vi "Get Main.Limitation.vi"(0 "Main":string="0", 1 "VI Ref":refnum<vi>, 2 "CMD":T2(ring)=enum."Read", 5 "Order By":T1, 9 "VariableName":string, 11 "error in (no error)":errorcluster, 12 "Alarm?":bool=TRUE) -> (3 "Unit":string, 4 "Data-DBL":cluster{"Max":dbl, "Min":dbl}, 6 "Data-String":cluster{"Max":string, "Min":string}, 10 "Limitation Table":string[](array[string]), 14 "Result Set":string[][](array[string]), 15 "error out":errorcluster)   [LabVIEW 2017, in "SQLite.lvclass"]
doc: "get Limitation Data.\n2015-11-03 10:56:51\n蒋松\njiangsong@outlook.com"
uses:
  SQLite.lvclass
  Order By.ctl
  SQLiteFileName.ctl
  TabelFullName.ctl
  <vilib>/Utility/error.llb/Trim Whitespace.vi
  <userlib>/LabSQL/LabSQL.lvlib
  <userlib>/sushu/sushu.lvlib
panel:
  out "Select SQL CMD":string
  # "Initialize\nRead\nWrite\nUnInitialize"
  # "TorqueAnglePrecision"
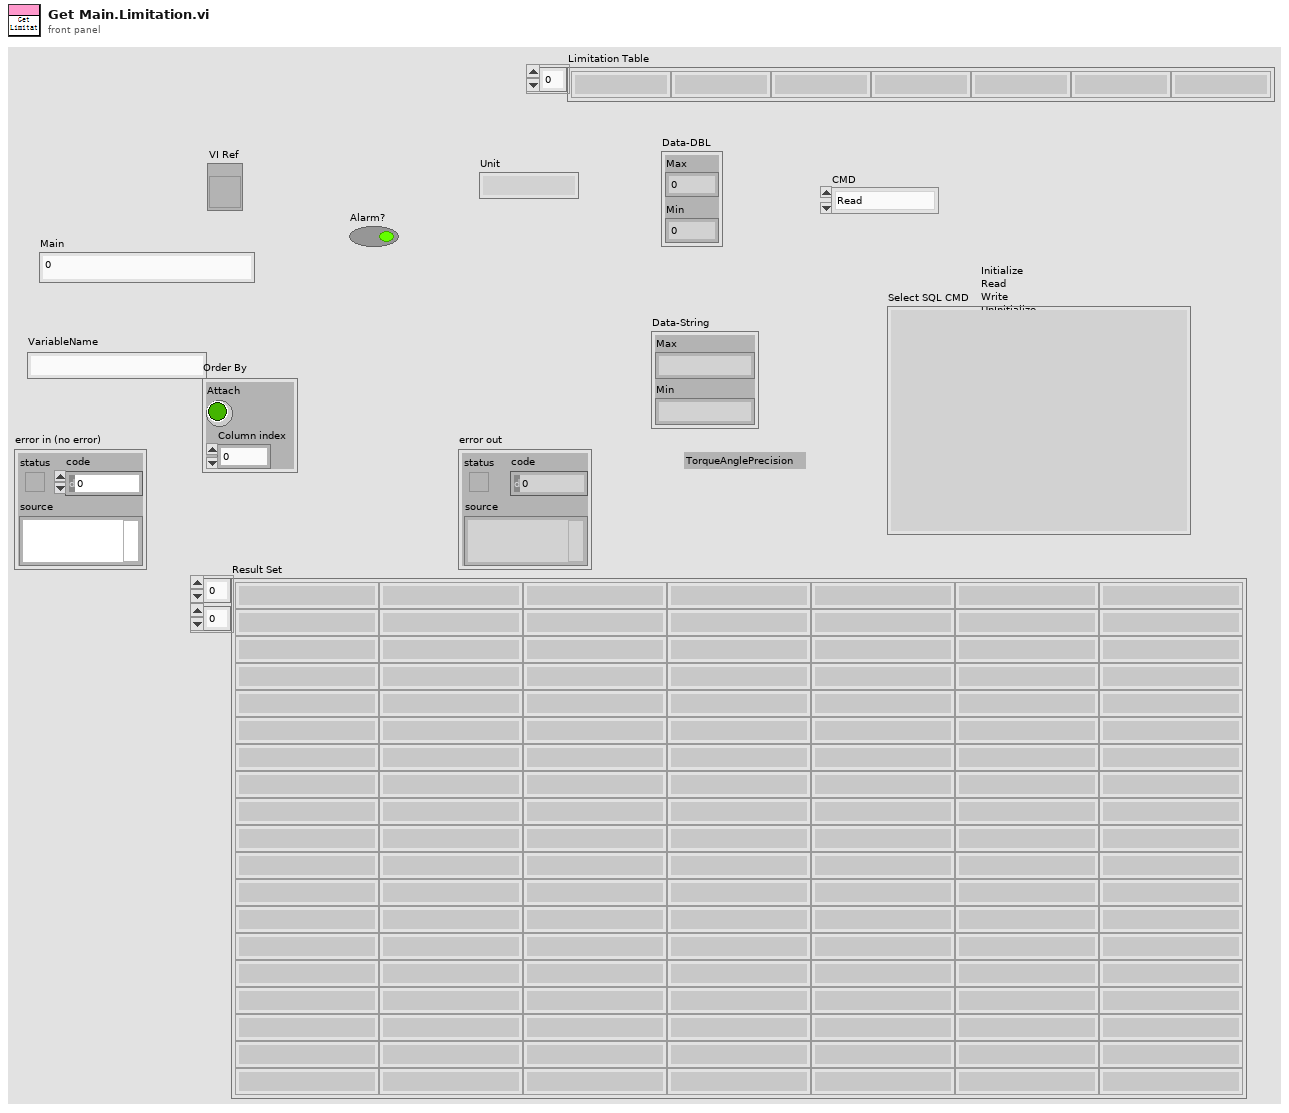
[diagram p1: front panel]
types:
  T1 = typedef "SQLite.lvclass/Order By.ctl" = cluster{"Attach":bool, "Column index":i32}
  T2 = enum16{"Initialize", "Read", "Write", "UnInitialize"}
  T3 = typedef "SQLite.lvclass/TabelFullName.ctl" = string
  T4 = typedef "SQLite.lvclass/SQLiteFileName.ctl" = string
  T5 = cluster{"Current VI Reference":refnum<vi>, "Close Panel on Exit?":bool}
  T6 = cluster{"Core":cluster{"Current VI Reference":refnum<vi>, "Close Panel on Exit?":bool}, "VI Name":string}
  T7 = enum32{"invalid app kind", "Development System", "Run Time System", "Student Edition", "Embedded LabVIEW", "Evaluation", "Custom"}
  T8 = enum32{"Invalid", "Standard", "Closed", "Hidden", "Minimized", "Maximized"}
  T9 = enum16{"Other", "SQL2008", "SQLite", "Access", "MySQL"}
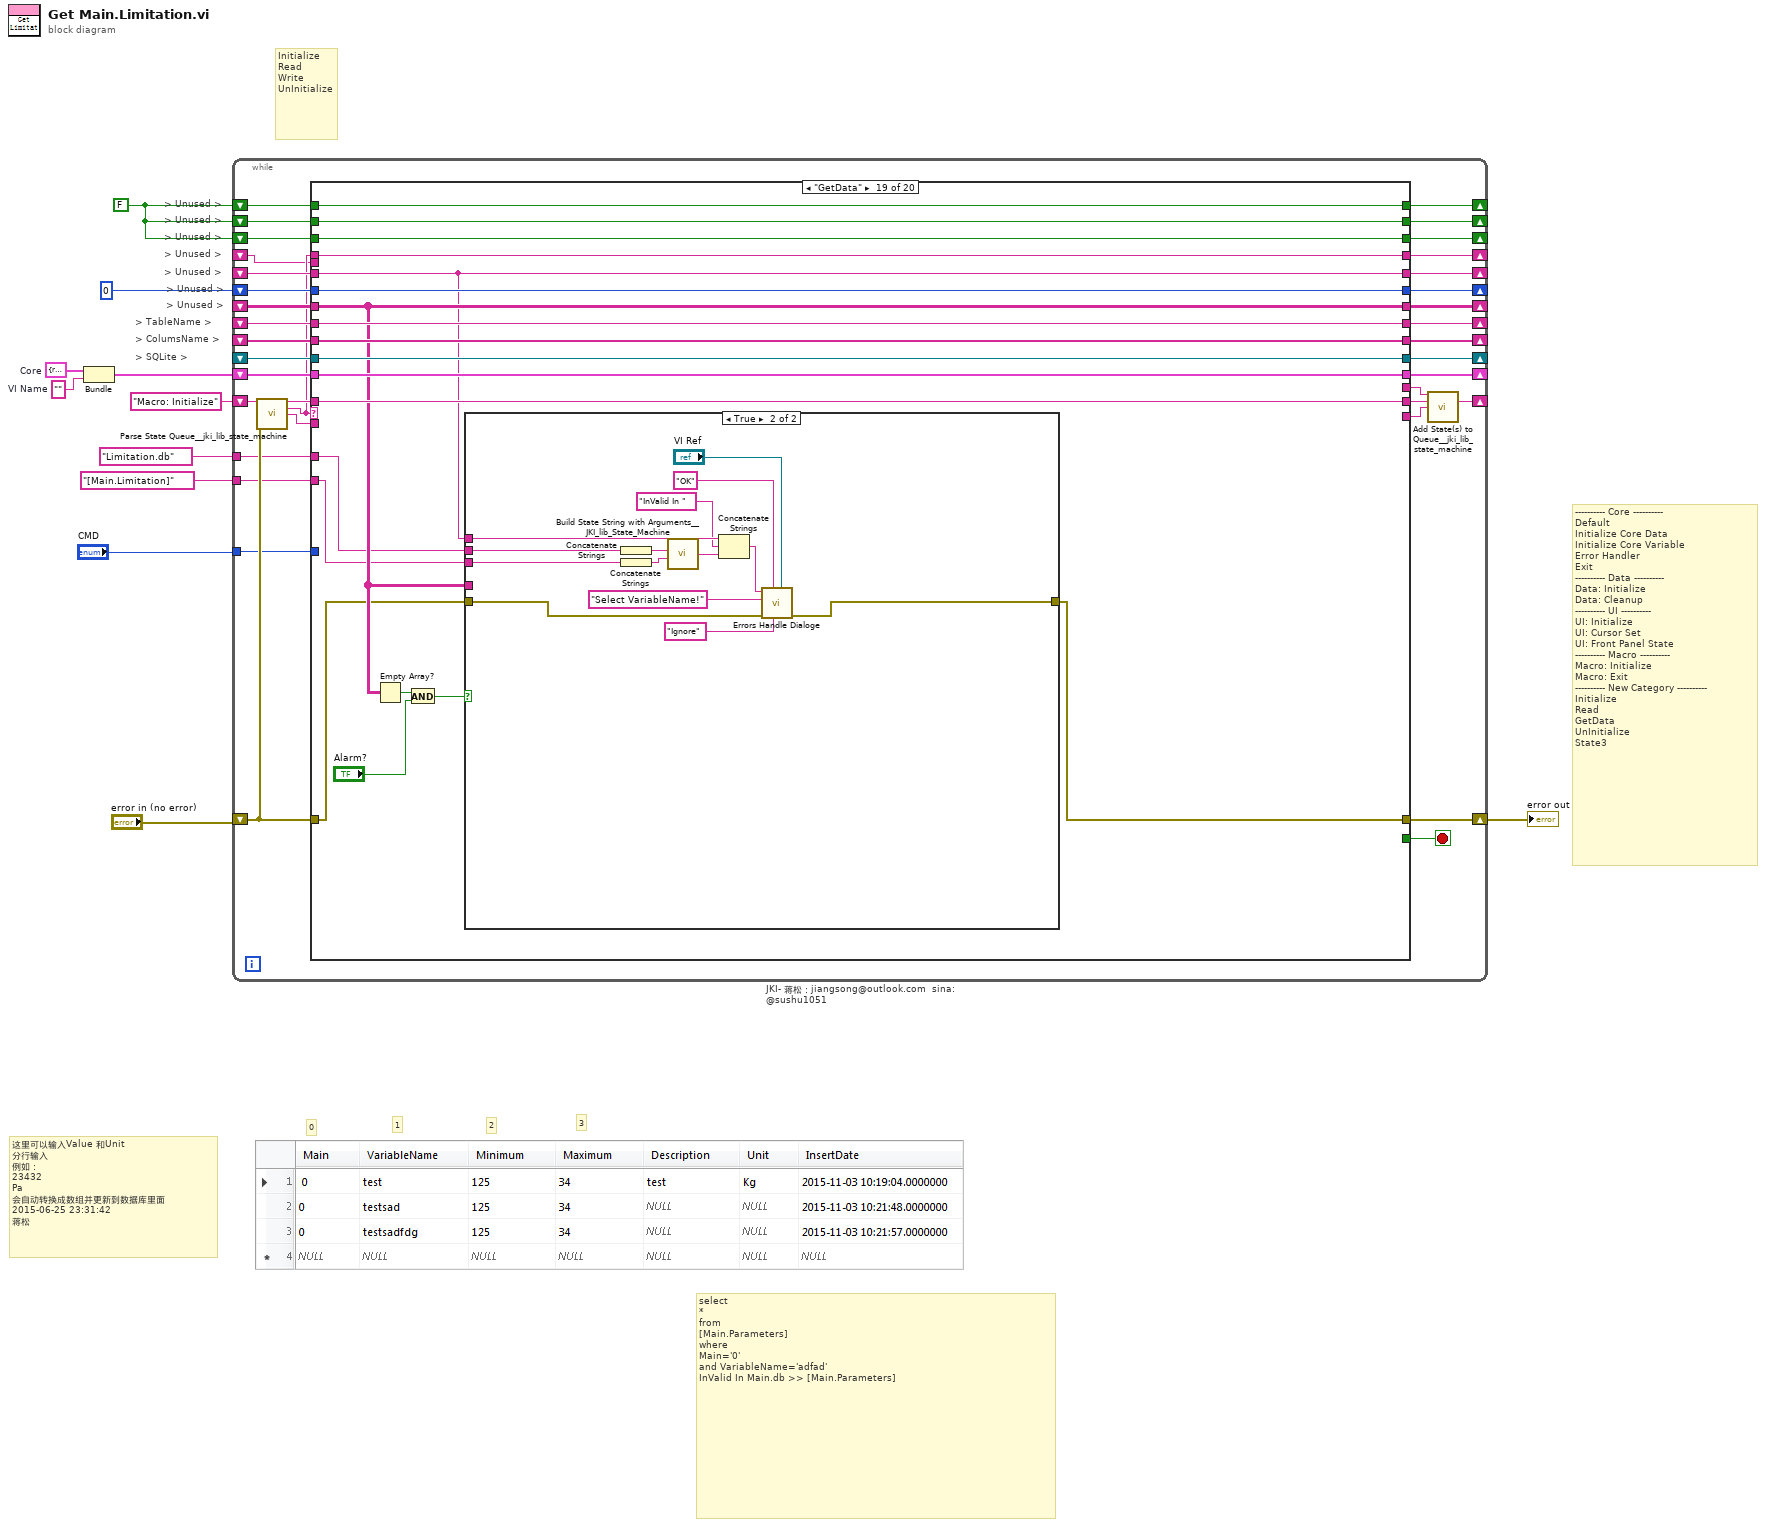
[diagram p0: block diagram]
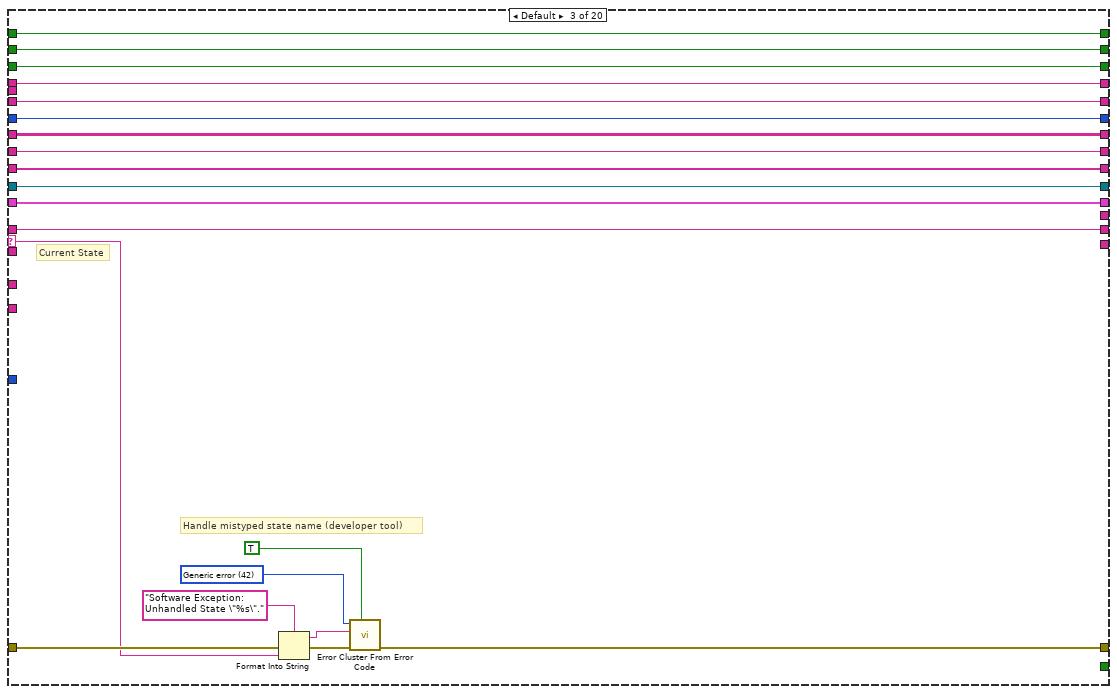
[diagram p4: hidden frame]
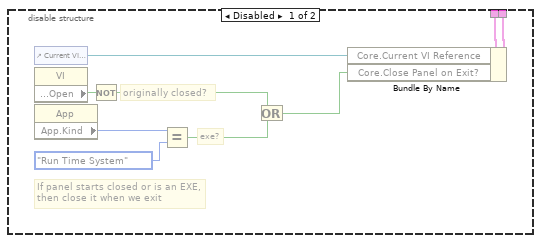
[diagram p6: hidden frame]
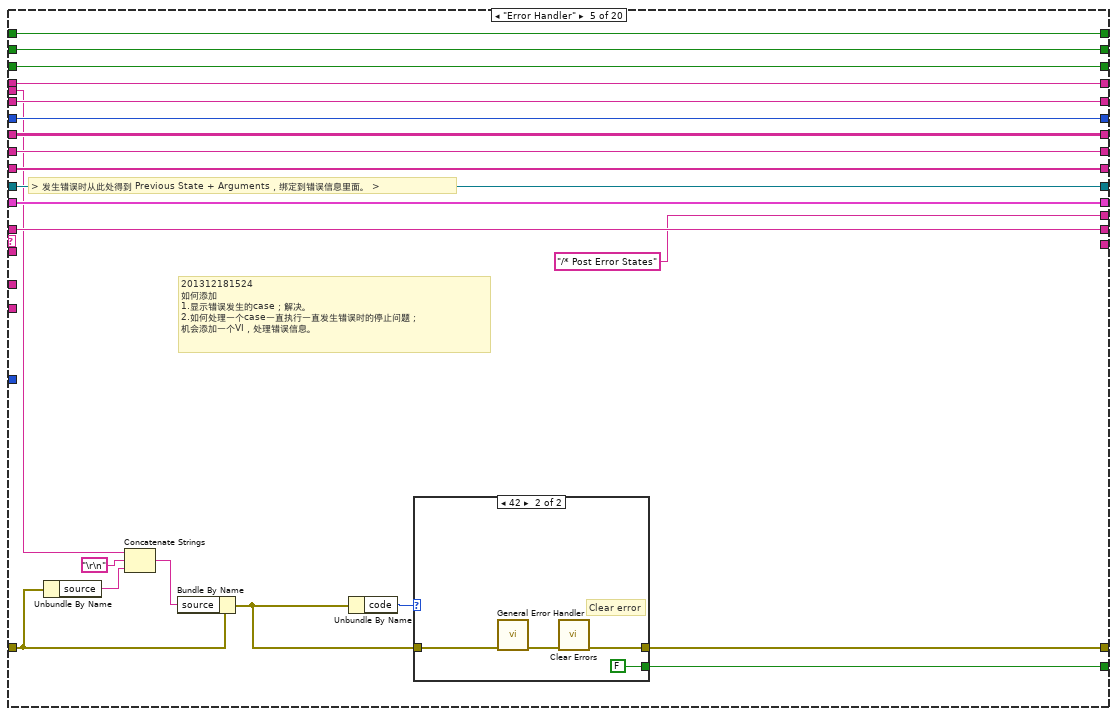
[diagram p7: hidden frame]
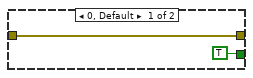
[diagram p8: hidden frame]
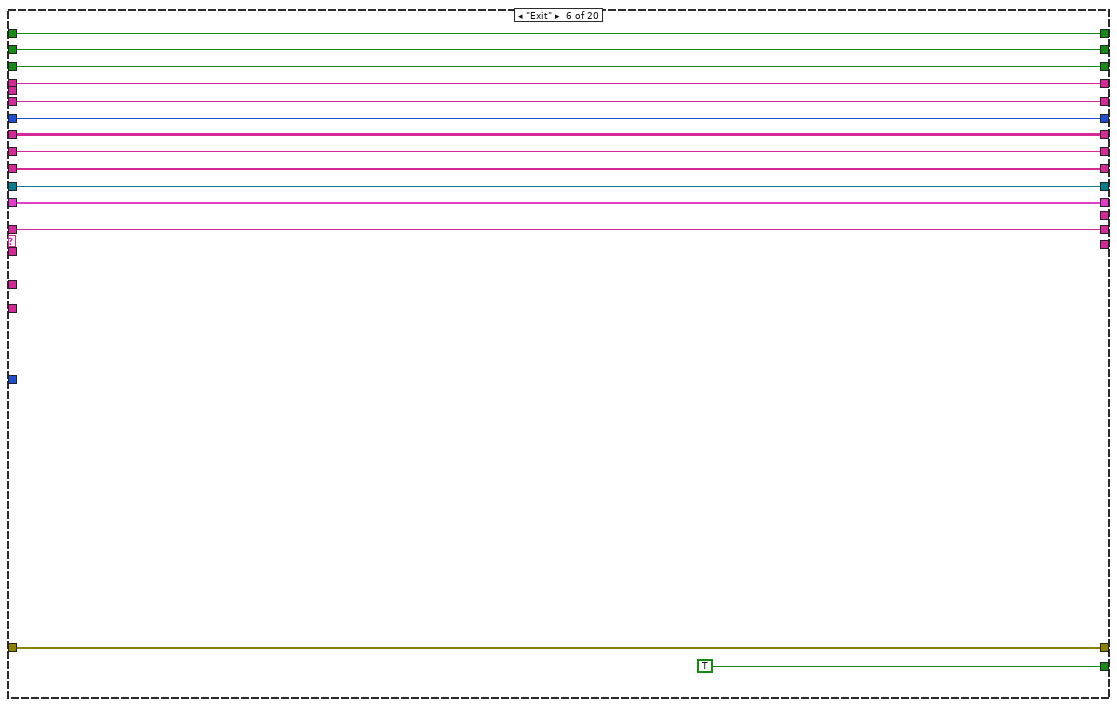
[diagram p9: hidden frame]
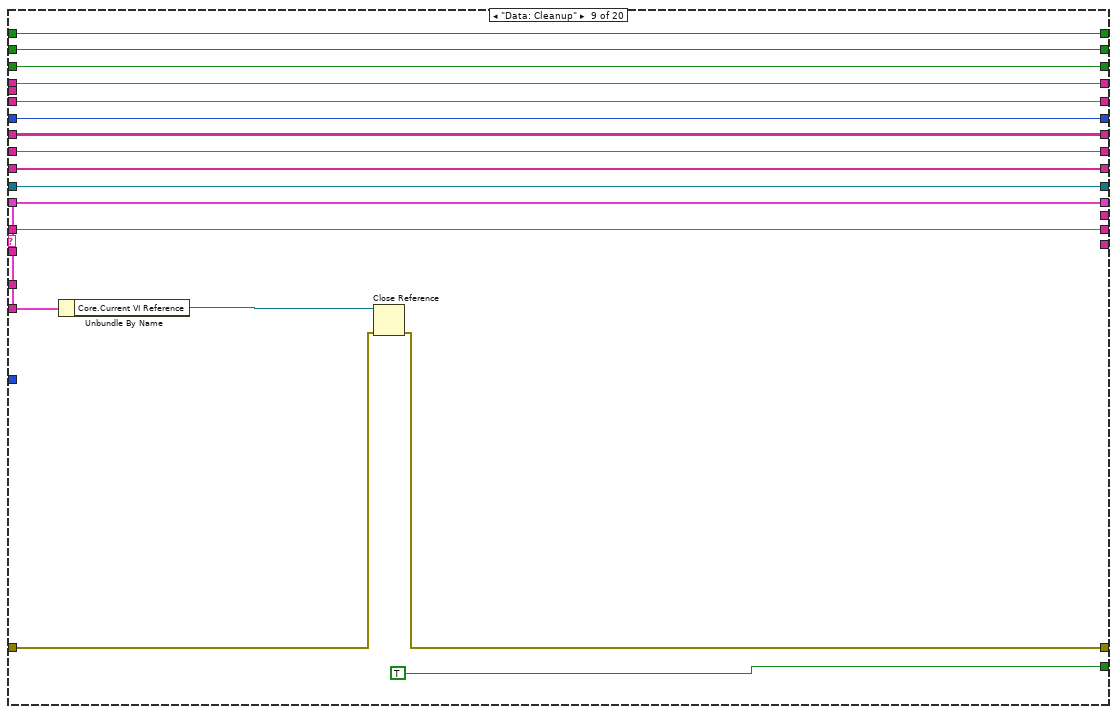
[diagram p12: hidden frame]
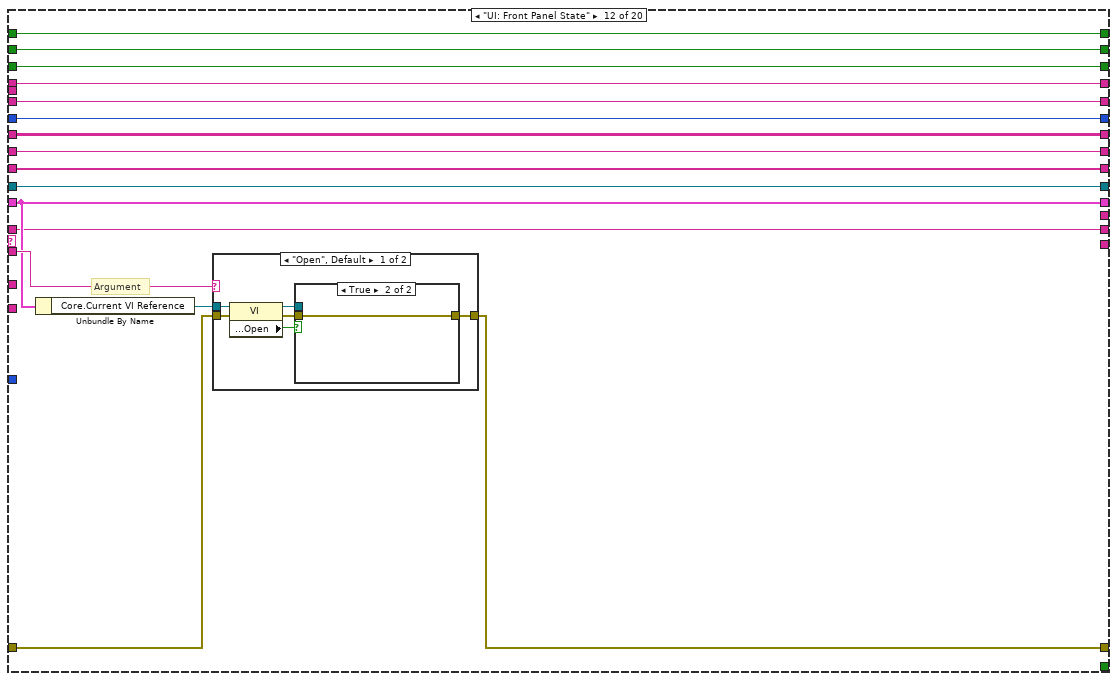
[diagram p15: hidden frame]
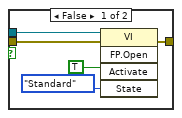
[diagram p16: hidden frame]
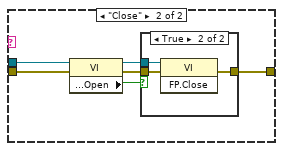
[diagram p17: hidden frame]
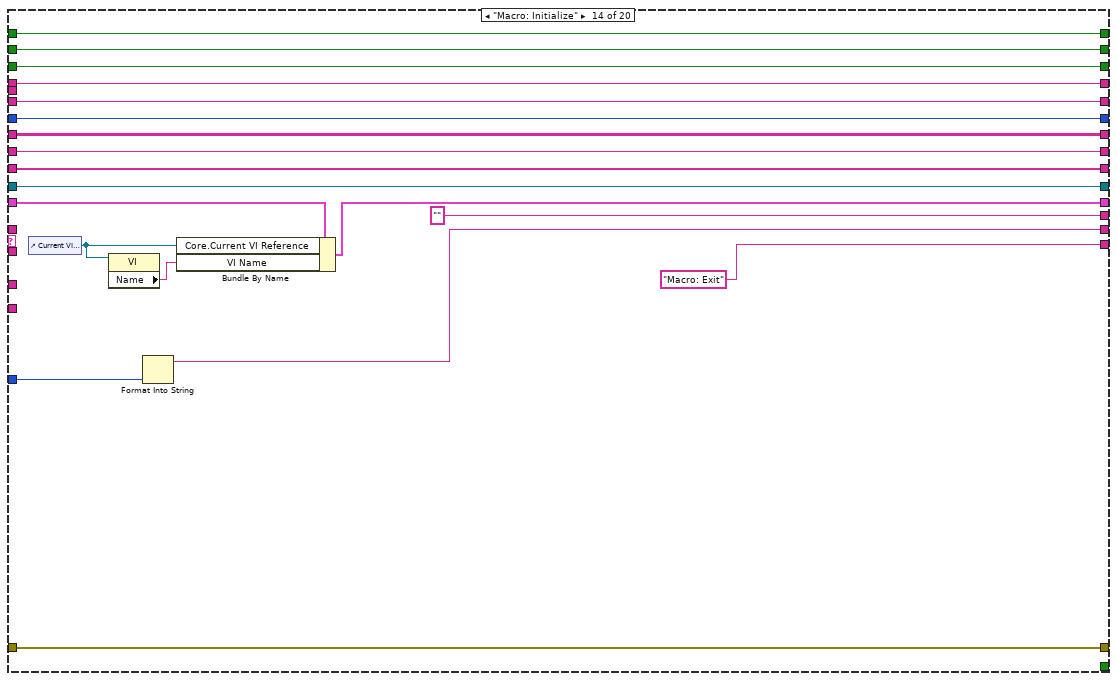
[diagram p20: hidden frame]
diagram:
  w11 = ""  # VI Name
  w10 = T5 {"Current VI Reference"=refnum, "Close Panel on Exit?"=FALSE}  # Core
  w3 = FALSE
  # "Initialize\nRead\nWrite\nUnInitialize"
  # "> Unused >"
  # "> Unused >"
  # "> Unused >"
  # "> Unused >"
  # "> Unused >"
  # "> Unused >"
  # "> SQLite >"
  # "> ColumsName >"
  # "> TableName >"
  # "> Unused >"
  # "---------- Core ----------\nDefault\nInitialize Core Data\nInitialize Core Variable\nError Handler\nExit\n---------- Data ----------\nData: Initialize\nData: Cleanup\n---------- UI ----------\nUI: Initialize\nUI: Cursor Set\nUI: Front Panel State\n---------- Macro ----------\nMacro: Initialize\nMacro: Exit\n---------- New Category ----------\nInitialize\nRead\nGetData\nUnInitialize\nState3"
  # "3"
  # "2"
  # "1"
  # "0"
  # "select\n*\nfrom\n[Main.Parameters]\nwhere\nMain='0'\nand VariableName='adfad'\nInValid In Main.db >> [Main.Parameters]"
  # "这里可以输入Value 和Unit\n分行输入\n例如：\n23432\nPa\n会自动转换成数组并更新到数据库里面\n2015-06-25 23:31:42\n蒋松"
  n1 = Bundle("Core"=w10, "VI Name"=w11) -> (w9:T6)  [unwired: 1 in]
  n2 = while "JKI- 蒋松：jiangsong@outlook.com  sina: @sushu1051" {
    shift-right: [w45] -> w5
    shift-left: "error in (no error)" -> [w43]
    shift-right: [w32] -> _
    shift-left: "Macro: Initialize" -> [w33]
    shift-right: [w39] -> _
    shift-left: _ -> [w41]
    shift-right: [w40] -> _
    shift-left: _ -> [w42]
    shift-right: [w34] -> _
    shift-left: w9 -> [w37]
    shift-right: [w35] -> _
    shift-left: _ -> [w28]
    shift-right: [w36] -> _
    shift-left: _ -> [w38]
    shift-right: [w27] -> _
    shift-left: 0 -> [w26]
    shift-right: [w20] -> _
    shift-left: w3 -> [w18]
    shift-right: [w19] -> _
    shift-left: w3 -> [w17]
    shift-right: [w22] -> _
    shift-left: _ -> [w23]
    shift-right: [w21] -> _
    shift-left: _ -> [w12]
    shift-right: [w24] -> _
    shift-left: w3 -> [w25]
    tunnel: "CMD" -> [w16]
    tunnel: T4 "Limitation.db" ("SQLiteFileName") -> [w15]
    tunnel: T3 "[Main.Limitation]" ("TabelFullName") -> [w14]
    stop <- w44 stop-if-true
    n3 = call <vilib>:"Parse State Queue__jki_lib_state_machine.vi"("State Queue"=w33, "Error In (no error)"=w43) -> ("Remaining States"=w47:string, "Current State"=w13:string, "Arguments"=w46:string)  [unwired: 10 in, 1 out]
    n4 = case shown="\"GetData\"" w13 {
      selector: w13 -> [_ _ w81 _ _ _ _ _ _ _ _ _ _ _ _ _ _ w358 _ _]
      tunnel: w47 -> [w60 w67 w80 w100 w131 w152 w166 w180 w193 w208 w221 w234 w272 _ w305 w322 w348 w383 w420 w469]
      tunnel: w46 -> [_ _ _ _ _ _ _ _ _ _ _ w237 _ _ _ _ _ _ _ _]
      tunnel: [w59 w73 w82 w104 w125 w154 w168 w182 w195 w210 w223 w238 w274 w294 w312 w325 w329 w353 w405 w455] -> w45
      tunnel: w43 -> [w59 w73 w83 w104 w135 w154 w168 w182 w196 w210 w223 w239 w274 w294 w312 w325 w329 w353 w406 w456]
      tunnel: [w60 w67 w80 w100 w131 w152 w166 w180 w193 w208 w221 w234 w272 w280 w305 w322 w348 w383 w420 w469] -> w31
      tunnel: [_ _ _ _ w124 TRUE _ _ TRUE _ _ _ _ _ _ _ _ _ _ _] -> w44
      tunnel: w42 -> [w58 w72 w93 w107 w139 w159 w172 w185 w201 w214 w227 w243 w278 w297 w315 w328 w347 _ w407 w468]
      tunnel: w41 -> [w57 w71 w92 w106 w138 w158 w171 w184 w200 w213 w226 w242 w277 w296 w314 w327 _ w363 w419 w467]
      tunnel: [w58 w72 w93 w107 w139 w159 w172 w185 w201 w214 w227 w243 w278 w297 w315 w328 w347 w354 w407 w468] -> w40
      tunnel: [w57 w71 w92 w106 w138 w158 w171 w184 w200 w213 w226 w242 w277 w296 w314 w327 w330 w363 w419 w467] -> w39
      tunnel: w38 -> [w56 w70 w91 w105 w137 w157 w170 w183 w199 w212 w225 w241 w276 w295 w313 w326 _ w364 w418 w466]
      tunnel: w28 -> [w54 w68 w90 w101 w129 w153 w167 w181 w194 w209 w222 w235 w273 w293 w306 w323 _ w357 w417 w458]
      tunnel: w37 -> [w55 w69 w89 w103 w136 w156 w169 w173 w197 w211 w224 w236 w275 w282 w307 w324 w346 w382 w416 w465]
      tunnel: [w56 w70 w91 w105 w137 w157 w170 w183 w199 w212 w225 w241 w276 w295 w313 w326 w332 w364 w418 w466] -> w36
      tunnel: [w54 w68 w90 w101 w129 w153 w167 w181 w194 w209 w222 w235 w273 w293 w306 w323 w334 w356 w417 w457] -> w35
      tunnel: [w55 w69 w89 w102 w136 w156 w169 w173 w197 w211 w224 w236 w275 w281 w307 w324 w346 w382 w416 w465] -> w34
      tunnel: [_ _ _ _ "/* Post Error States" _ _ _ _ _ _ _ _ "" w304 _ _ w360 _ _] -> w30
      tunnel: [_ _ _ _ _ _ _ _ _ _ _ _ _ "Macro: Exit" _ _ _ _ _ _] -> w29
      tunnel: w26 -> [w53 w66 w79 w99 w128 w151 w165 w179 w192 w207 w220 w233 w271 w292 w303 w321 w345 w361 w415 w464]
      tunnel: [w53 w66 w79 w99 w128 w151 w165 w179 w192 w207 w220 w233 w271 w292 w303 w321 w345 w362 w415 w464] -> w27
      tunnel: w17 -> [w51 w64 w77 w97 w122 w149 w163 w177 w190 w205 w218 w231 w269 w288 w301 w319 w340 w380 w414 w463]
      tunnel: w18 -> [w50 w63 w76 w96 w121 w148 w162 w176 w189 w204 w217 w230 w268 w287 w300 w318 w341 w379 w413 w462]
      tunnel: [w51 w64 w77 w97 w122 w149 w163 w177 w190 w205 w218 w231 w269 w288 w301 w319 w340 w380 w414 w463] -> w19
      tunnel: [w50 w63 w76 w96 w121 w148 w162 w176 w189 w204 w217 w230 w268 w287 w300 w318 w341 w379 w413 w462] -> w20
      tunnel: w13 -> [w49 w62 w75 w95 w120 w147 w161 w175 w188 w203 w216 w229 w267 w286 w299 w317 w342 w378 w412 w461]
      tunnel: w23 -> [w48 w61 w74 w94 w119 w146 w160 w174 w187 w202 w215 w228 w266 w285 w298 w316 w343 _ w402 w460]
      tunnel: [w49 w62 w75 w95 w120 w147 w161 w175 w188 w203 w216 w229 w267 w286 w299 w317 w342 w378 w412 w461] -> w21
      tunnel: [w48 w61 w74 w94 w119 w146 w160 w174 w187 w202 w215 w228 w266 w285 w298 w316 w343 w355 w402 w460] -> w22
      tunnel: w25 -> [w52 w65 w78 w98 w123 w150 w164 w178 w191 w206 w219 w232 w270 w289 w302 w320 w344 w381 w411 w459]
      tunnel: [w52 w65 w78 w98 w123 w150 w164 w178 w191 w206 w219 w232 w270 w289 w302 w320 w344 w381 w411 w459] -> w24
      tunnel: w16 -> [_ _ _ _ _ _ _ _ _ _ _ _ _ w279 _ _ _ _ _ _]
      tunnel: w15 -> [_ _ _ _ _ _ _ _ _ _ _ _ _ _ _ _ w333 _ w404 _]
      tunnel: w14 -> [_ _ _ _ _ _ _ _ _ _ _ _ _ _ _ _ w331 _ w403 _]
      tunnel: w12 -> [_ _ _ _ w118 _ _ _ _ _ _ _ _ _ _ _ _ _ _ _]
      frame "Idle" {
      }
      frame "---------- Core ----------" {
      }
      frame Default {
        w85 = 42 items=["No error", "Argument error", "Memory is full", "Out of zone", "End of file", "File already open", "Generic file I/O error", "File not found", "File permission error", "Disk is full", "Duplicate path", "Too many files open", "System feature not enabled", "Resource file not found", "Cannot add resource", "Resource not found", "Image not found", "Image memory error", "Pen does not exist", "Config type invalid", "Config token not found", "Config parse error", "Config memory error", "Bad external code format", "Bad external code offset", "External code not present", "Null window", "Destroy window error", "Null menu", "Print aborted", "Bad print record", "Print driver error", "Windows error during printing", "Memory error during printing", "Print dialog error", "Generic print error", "Invalid device refnum", "Device not found", "Device parameter error", "Device unit error", "Cannot open device", "Device call aborted", "Generic error", "Cancelled by user", "Object ID too low", "Object ID too high", "Object not in heap", "Unknown heap", "Unknown object (invalid DefProc)", "Unknown object (DefProc not in table)", "Message out of range", "Invalid (null) method", "Unknown message", "Manager call not supported", "Bad address", "Network operation in progress", "Network operation timed out", "Connection is busy", "Network attribute not supported", "Network error", "Address in use", "System out of memory", "Connection aborted", "Connection refused", "Not connected", "Already connected", "Connection closed", "Initialization error (interapplication manager)", "Bad occurrence", "Wait on unbound occurrence handler", "Occurrence queue overflow", "Datalog type conflict", "Unused", "Unrecognized type (interapplication manager)", "Memory corrupt", "Failed to make temporary DLL", "Old CIN version", "Drag socket not found", "Failed to load drop-object", "Failed to register OLE object", "Failed to release OLE object", "Format specifier type mismatch", "Unknown format specifier", "Too few format specifiers", "Too many format specifiers", "Scan failed", "Newer CIN version", "Error converting to variant", "Runtime menu error", "Password tampered", "Variant attribute not found", "Incompatible variant data type", "Event data is not available", "Event Store is not present", "Occurrence is not found", "Event Queue is not created", "Event info is not available", "Refnum passed is NULL", "Error retrieving Class GUID", "Error retrieving CoClass GUID", "Error retrieving TypeLib GUID.", "Bad built application magic bytes.", "Specific driver is different from the specific driver associated with the Logical Name.", "There is no session opened to the class driver.", "Max Error", "MAX - Error with config objects", "MAX - Error loading configuration", "MAX - Group not supported"]
        # "Current State"
        # "Handle mistyped state name (developer tool)"
        n5 = Format Into String(format string="Software Exception: Unhandled State \"%s\"." ("message"), error in=w83, w81) -> (resulting string=w86:string, error out=w87:errorcluster)  [unwired: 1 in]
        n6 = call <vilib>:"Error Cluster From Error Code.vi"("show call chain? (False)"=TRUE, "error in (no error)"=w87, "error message (\"\")"=w86, "error code (0)"=w85) -> ("error out"=w82:errorcluster)  [unwired: 5 in]
      }
      frame "Initialize Core Data" {
        n7 = disable-structure shown="Enabled" {
          disable-tunnel: w103 -> [w109 w117]
          disable-tunnel: [w108 w117] -> w102
          frame Disabled {
            # "originally closed?"
            # "exe?"
            # "If panel starts closed or is an EXE, then close it when we exit"
            n8 = control-ref of="Current VI Reference"() -> (w116:refnum<vi>)
            n9 = property class="VI"() -> ("Front Panel.Open"=w110:bool)  [unwired: 2 in, 2 out]
            n10 = property class="App"() -> ("App.Kind"=w111:T7)  [unwired: 2 in, 2 out]
            n11 = Not(x=w110) -> (.not. x?=w113:bool)
            n12 = Equal?(x=w111, y=T7."Run Time System" ("Application:Kind")) -> (x = y?=w114:bool)
            n13 = Or(x=w113, y=w114) -> (x .or. y?=w115:bool)
            n14 = Bundle By Name(cluster=w109, "Core.Current VI Reference"=w116, "Core.Close Panel on Exit?"=w115) -> (w108:T6)
          }
          frame Enabled {
          }
        }
      }
      frame "Error Handler" {
        # "> 发生错误时从此处得到 Previous State + Arguments，绑定到错误信息里面。 >"
        # "201312181524\n如何添加\n1.显示错误发生的case；解决。\n2.如何处理一个case一直执行一直发生错误时的停止问题；\n机会添加一个VI，处理错误信息。"
        # "Clear error"
        n15 = Unbundle By Name(w135) -> ("source"=w133:string)
        n16 = Concatenate Strings(w118, "\r\n", w133) -> (w132:string)
        n17 = Bundle By Name(cluster=w135, "source"=w132) -> (w126:errorcluster)
        n18 = Unbundle By Name(w126) -> ("code"=w127:i32)
        n19 = case shown="42" w127 {
          tunnel: [TRUE FALSE] -> w124
          tunnel: w126 -> [w141 w144]
          tunnel: [w141 w142] -> w125
          frame 0, Default {
          }
          frame 42 {
            n20 = call <vilib>:"General Error Handler.vi"("error in (no error)"=w144) -> ("error out"=w143:errorcluster)  [unwired: 10 in, 4 out]
            n21 = call <vilib>:"Clear Errors.vi"("error in (no error)"=w143) -> ("error out"=w142:errorcluster)  [unwired: 5 in, 1 out]
          }
        }
      }
      frame "Exit" {
      }
      frame "---------- Data ----------" {
      }
      frame "Data: Initialize" {
      }
      frame "Data: Cleanup" {
        n22 = Unbundle By Name(w197) -> ("Core.Current VI Reference"=w198:refnum<vi>)
        n23 = Close Reference(reference=w198, error in (no error)=w196) -> (error out=w195:errorcluster)
      }
      frame "---------- UI ----------" {
      }
      frame "UI: Initialize" {
      }
      frame "UI: Front Panel State" {
        # "Argument"
        n24 = Unbundle By Name(w236) -> ("Core.Current VI Reference"=w240:refnum<vi>)
        n25 = case shown="\"Open\", Default" w237 {
          tunnel: w239 -> [w247 w260]
          tunnel: [w249 w261] -> w238
          tunnel: w240 -> [w248 w258]
          frame "Open", Default {
            n26 = property class="VI"(reference=w248, error in=w247) -> (reference out=w245:refnum<vi>, error out=w246:errorcluster, "Front Panel.Open"=w244:bool)
            n27 = case shown="True" w244 {
              tunnel: [w252 w255] -> w249
              tunnel: w246 -> [w251 w255]
              tunnel: w245 -> [w250 _]
              frame False {
                n28 = invoke class="VI" method="FP.Open"(reference=w250, error in=w251, "Activate"=TRUE, "State"=T8."Standard") -> (error out=w252:errorcluster)  [unwired: 1 in, 4 out]
              }
              frame True {
              }
            }
          }
          frame "Close" {
            n29 = property class="VI"(reference=w258, error in=w260) -> (reference out=w257:refnum<vi>, error out=w259:errorcluster, "Front Panel.Open"=w256:bool)
            n30 = case shown="True" w256 {
              tunnel: [w262 w265] -> w261
              tunnel: w259 -> [w262 w264]
              tunnel: w257 -> [_ w263]
              frame False {
              }
              frame True {
                n31 = invoke class="VI" method="FP.Close"(reference=w263, error in=w264) -> (error out=w265:errorcluster)  [unwired: 1 in, 2 out]
              }
            }
          }
        }
      }
      frame "---------- Macro ----------" {
      }
      frame "Macro: Initialize" {
        n32 = control-ref of="Current VI Reference"() -> (w283:refnum<vi>)
        n33 = property class="VI"(reference=w283) -> ("Name"=w284:string)  [unwired: 1 in, 2 out]
        n34 = Format Into String(w279) -> (resulting string=w280:string)  [unwired: 3 in, 1 out]
        n35 = Bundle By Name(cluster=w282, "Core.Current VI Reference"=w283, "VI Name"=w284) -> (w281:T6)
      }
      frame "Macro: Exit" {
        n36 = Unbundle By Name(w307) -> ("Core.Close Panel on Exit?"=w308:bool)
        n37 = Select(t="UI: Front Panel State >> Close", s=w308, f="") -> ()  [unwired: 1 out]
        n38 = call <vilib>:"Add State(s) to Queue__jki_lib_state_machine.vi"("State(s) at Back (\"\")"="Data: Cleanup\nExit") -> ("States Out"=w304:string)  [unwired: 14 in]
      }
      frame "---------- New Category ----------" {
      }
      frame "Initialize" {
        n39 = Concatenate Strings(w331) -> (w330:string)
        n40 = call "SQLite File Path.vi"("SQLiteFileName"=w333, "SQLite in"=refnum<class "SQLite.lvclass"> refnum ("SQLite.lvclass")) -> ("string"=w337:string, "SQLite out"=w339:refnum<class "SQLite.lvclass">)  [unwired: 7 in, 1 out]
        n41 = call-dynamic "Open Connection.vi"("ConnectionString"=w337, "HostDB in"=w339) -> ("error out"=w336:errorcluster, "HostDB out"=w335:refnum<class "SQLite.lvclass">)  [unwired: 8 in]
        n42 = call-dynamic "Get Table Columns Name.vi"("error in (no error)"=w336, "TableName"=w330, "HostDB in"=w335) -> ("ColunmsList"=w332:string[], "HostDB out"=w334:refnum<class "SQLite.lvclass">)  [unwired: 4 in, 3 out]
      }
      frame "Read" {
        n43 = Empty String/Path?(string/path="VariableName") -> (empty?=w375:bool)
        n44 = Unbundle By Name("Order By") -> ("Attach"=w368:bool, "Column index"=w367:i32)
        n45 = Build Array("Main") -> (w371:string[])
        n46 = Build Array("Main", "VariableName") -> (w373:string[])
        n47 = Select(t=w371, s=w375, f=w373) -> (s? t:f=w370:string[])
        n48 = Array Size(array=w370) -> (size(s)=w369:i32)
        n49 = Array Subset(array=w364, index=0, length=w369) -> (w377:string[])
        n50 = Index Array(array=w364, index=w367) -> (element=w366:string)
        n51 = call <userlib>:"SQL_Select From DB Table.vi"("DB Type"=T9."SQLite", "ColumnsValue"=w370, "ColumnsNameList"=w377, "TableName"=w363) -> ("Select SQL CMD"=w365:string)  [unwired: 7 in]
        "Select SQL CMD" <- w365
        n52 = case shown="True" w368 {
          tunnel: w365 -> [w395 w400]
          tunnel: w366 -> [_ w398]
          tunnel: [w395 w396] -> w355
          frame False {
          }
          frame True {
            n53 = Concatenate Strings(w400, "\r", "order by cast (" ("string"), w398, " as unsigned)" ("string")) -> (w396:string)
          }
        }
        n54 = call-dynamic "SQL Execute.vi"("error in (no error)"=w353, "Return Data (T)"=TRUE, "Command Text"=w355, "HostDB in"=w357) -> ("error out"=w352:errorcluster, "Table Control"=w354:string[][], "HostDB out"=w356:refnum<class "SQLite.lvclass">)  [unwired: 3 in, 2 out]
        n55 = case shown="Error" w352 {
          tunnel: w352 -> [_ w394]
          tunnel: w361 -> [_ w393]
          tunnel: [w384 w390] -> w360
          tunnel: "GetData" ("f") -> [w384 w389]
          tunnel: w358 -> [_ w386]
          frame No Error {
          }
          frame Error {
            (unwired) 7 ("y")
            n56 = Unbundle By Name(w394) -> ("status"=w385:bool)
            n57 = Equal To 0?(x=w393) -> (x = 0?=w392:bool)
            n58 = And(x=w385, y=w392) -> (x .and. y?=w391:bool)
            n59 = call <vilib>:"Add State(s) to Queue__jki_lib_state_machine.vi"("State(s) in Front (\"\")"="Initialize" ("Remaining States"), "State(s) in (\"\")"=w386) -> ("States Out"=w387:string)  [unwired: 13 in]
            n60 = Select(t=w387, s=w391, f=w389) -> (s? t:f=w390:string)
          }
        }
        n61 = Increment(x=w361) -> (x+1=w362:i32)
      }
      frame "GetData" {
        n62 = Empty Array?(array=w407) -> (empty?=w409:bool)
        n63 = And(x=w409, y="Alarm?") -> (x .and. y?=w410:bool)
        n64 = case shown="True" w410 {
          tunnel: [w440 w453] -> w405
          tunnel: w406 -> [w440 w454]
          tunnel: w402 -> [_ w450]
          tunnel: w404 -> [_ w452]
          tunnel: w403 -> [_ w451]
          tunnel: w407 -> [w431 _]
          frame False {
            w428 = cluster{"Max":dbl, "Min":dbl} {"Max"=0.0, "Min"=0.0}  # Data-DBL
            w430 = cluster{"Max":string, "Min":string} {"Max"="", "Min"=""}  # Data-String
            # "DBL 和 字符串 都输出，需要那个用那个。\n2015-11-03 10:44:12\n蒋松"
            n65 = Array Size(array=w431) -> (size(s)=w439:i32[])
            n66 = Index Array(array=w439) -> (element #2=w438:i32)  [unwired: 2 in, 1 out]
            n67 = Decrement(x=w438) -> (x-1=w437:i32)
            n68 = Delete From Array(array=w431, length=1 ("disabled index (col)"), index (col)=w437) -> (array with subset deleted=w434:string[][])  [unwired: 1 in, 1 out]
            n69 = Index Array(array=w434, index (row)=0) -> (element=w433:string[])  [unwired: 1 in]
            n70 = Array Subset(array=w433, index=2) -> (w422:string[])  [unwired: 1 in]
            "Limitation Table" <- w422
            n71 = Index Array(array=w422) -> (element #1=w429:string, element #2=w426:string, element #3=→"Unit":string)  [unwired: 3 in]
            n72 = Fract/Exp String To Number(string=w429) -> (number=w427:dbl)  [unwired: 3 in, 1 out]
            n73 = Fract/Exp String To Number(string=w426) -> (number=w425:dbl)  [unwired: 3 in, 1 out]
            n74 = Bundle By Name(cluster=w430, "Min"=w429, "Max"=w426) -> (→"Data-String":cluster{"Max":string, "Min":string})
            n75 = Bundle By Name(cluster=w428, "Min"=w427, "Max"=w425) -> (→"Data-DBL":cluster{"Max":dbl, "Min":dbl})
            "Result Set" <- w431
          }
          frame True {
            n76 = Concatenate Strings(w452) -> (w449:string)
            n77 = Concatenate Strings(w451) -> (w448:string)
            n78 = call <vilib>:"Build State String with Arguments__JKI_lib_State_Machine.vi"("Arguments (\"\")"=w448, "State"=w449) -> ("State with Arguments"=w446:string)  [unwired: 4 in]
            n79 = Concatenate Strings(w450, "InValid In " ("Message"), w446) -> (w445:string)
            n80 = call <userlib>:"Errors Handle Dialoge.vi"("VI Ref"="VI Ref", "Cancel Text"="Ignore", "OK Text"="OK", "error in (no error)"=w454, "Title Text"="Select VariableName!", "Message"=w445) -> ("error out"=w453:errorcluster)  [unwired: 4 in, 1 out]
          }
        }
      }
      frame "UnInitialize" {
        n81 = call-dynamic "Close Connection.vi"("error in (no error)"=w456, "HostDB in"=w458) -> ("error out"=w455:errorcluster, "HostDB out"=w457:refnum<class "SQLite.lvclass">)  [unwired: 8 in]
      }
    }
    n82 = call <vilib>:"Add State(s) to Queue__jki_lib_state_machine.vi"("State(s) in Front (\"\")"=w30, "State(s) in (\"\")"=w31, "State(s) at Back (\"\")"=w29) -> ("States Out"=w32:string)  [unwired: 12 in]
  }
  "error out" <- w5
